vi "Begin.vi"(8 "error in":errorcluster) -> (0 "error out":errorcluster)   [LabVIEW 2016]
doc: "Called before other user functions, this VI is expected to open initial I/O refnums, load in file data, and do all program initialization. Notice that the <B>error out</B> terminal is simply used for data flow. Wiring it to other structures or subVIs ensures that this VI runs first."
uses:
  <vilib>/Rock Robotics/SystemInterfaces/DIO/FPGA_DIOPWMChannel.ctl
  <vilib>/Rock Robotics/WPI/SafetyOutput/WPI_SafetyOutputConfigMenu.ctl
  <vilib>/Rock Robotics/WPI/DriverStation/WPI_DriverStationRobotMode2.ctl
  <vilib>/Rock Robotics/WPI/Joystick/WPI_JoystickDeviceEnum.ctl
  <vilib>/Rock Robotics/SystemInterfaces/DIO/FPGA_DIOChannel.ctl
  <vilib>/Rock Robotics/WPI/RobotDrive/WPI_RobotDriveOpen2MotorWithTalon.vi
  Robot Global Data.vi
  <vilib>/Rock Robotics/Network Tables/NT Write String Array.vi
  <vilib>/Rock Robotics/WPI/Ultrasonic/WPI_SonarSRF04DigitalOpen.vi
  <vilib>/Rock Robotics/WPI/Ultrasonic/WPI_SonarSRF04DigitalRefNum Registry Set.vi
  Globals/Globals.vi
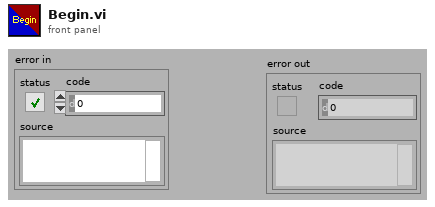
[diagram p1: front panel]
types:
  T1 = typedef "FPGA_DIOChannel.ctl" = enum8{"DIO 0", "DIO 1", "DIO 2", "DIO 3", "DIO 4", "DIO 5", "DIO 6", "DIO 7", "DIO 8", "DIO 9", "DIO MXP 0", "DIO MXP 1", "DIO MXP 2", "DIO MXP 3", "DIO MXP 4", "DIO MXP 5", "DIO MXP 6", "DIO MXP 7", "DIO MXP 8", "DIO MXP 9", "DIO MXP 10", "DIO MXP 11", "DIO MXP 12", "DIO MXP 13", "DIO MXP 14", "DIO MXP 15", "SPI Port CS1", "SPI Port CS2", "SPI Port CS3", "SPI Port MISO", "SPI Port MOSI", "Invalid"}
  T2 = typedef "FPGA_DIOPWMChannel.ctl" = enum8{"PWM 0", "PWM 1", "PWM 2", "PWM 3", "PWM 4", "PWM 5", "PWM 6", "PWM 7", "PWM 8", "PWM 9", "PWM MXP 0", "PWM MXP 1", "PWM MXP 2", "PWM MXP 3", "PWM MXP 4", "PWM MXP 5", "PWM MXP 6", "PWM MXP 7", "PWM MXP 8", "PWM MXP 9", "Invalid"}
  T3 = typedef "WPI_JoystickDeviceEnum.ctl" = enum16{"USB 0", "USB 1", "USB 2", "USB 3", "USB 4", "USB 5"}
  T4 = typedef "WPI_DriverStationRobotMode2.ctl" = enum16{"Autonomous Disabled", "Autonomous Enabled", "Teleop Disabled", "Teleop Enabled", "Disconnected", "Finish", "Test Disabled", "Test Enabled", "Emergency Stopped"}
  T5 = typedef "WPI_SafetyOutputConfigMenu.ctl" = enum16{"Enable", "Disable"}
  T6 = typedef "WPI_UltrasonicDeviceRef.ctl" = cluster{"DevStatus":errorcluster, "Ping Channel":T1, "Echo Channel":T1, "CntIndex":T7}
  T7 = typedef "FPGA_CounterCtrSystemIndex.ctl" = enum8{"Ctr 0", "Ctr 1", "Ctr 2", "Ctr 3", "Ctr 4", "Ctr 5", "Ctr 6", "Ctr 7", "Invalid"}
  T8 = typedef "WPI_JoystickDevRef.ctl" = cluster{"Device":T3}
  T9 = typedef "WPI_RobotDriveDevRef.ctl" = cluster{"DevStatus":errorcluster, "Motors[]":T10[], "Square Inputs":bool, "Max Output":dbl}
  T10 = typedef "WPI_MotorControlDeviceRef.ctl" = cluster{"DeviceStatus":errorcluster, "Type":T11, "PWM":cluster{"PWM Channel":T2, "DeadBand":T12}, "CAN":cluster{"Device Number":u8, "SetOutput VI Ref":variant, "GetOutput VI Ref":variant, "Enable VI Ref":variant, "Disable VI Ref":variant, "Data":variant}, "Invert":bool}
  T11 = typedef "WPI_MotorControlType.ctl" = enum16{"PWM", "CAN"}
  T12 = typedef "WPI_PWMDeadband.ctl" = cluster{"Name":string, "maxPositivePwm":i32, "minPositivePwm":i32, "centerPwm":i32, "maxNegativePwm":i32, "minNegativePwm":i32, "angularRange":u16}
  T13 = typedef "WPI_ServoDeviceRef.ctl" = cluster{"DeviceStatus":errorcluster, "PWM Channel":T2, "DeadBand":T12}
  T14 = typedef "WPI_DigitalOutputDevRef.ctl" = cluster{"DIO Channel":T1, "DevStatus":errorcluster}
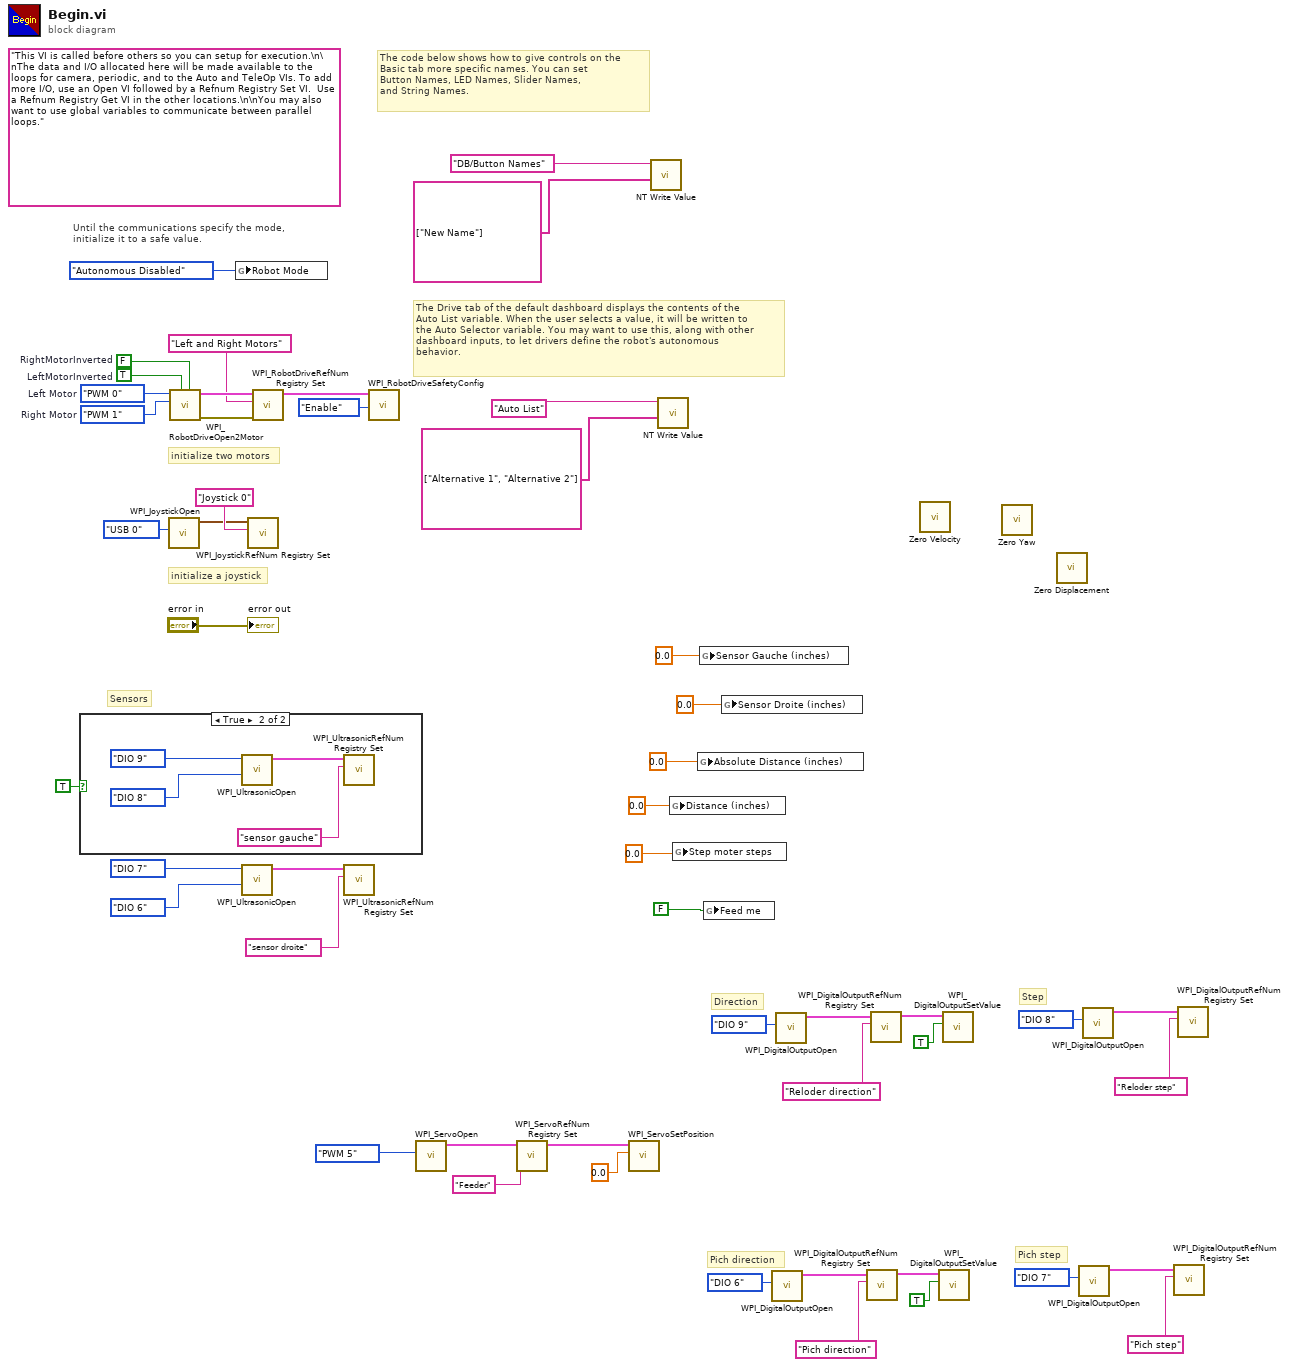
[diagram p0: block diagram]
diagram:
  (unwired) "This VI is called before others so you can setup for execution.\n\nThe data and I/O allocated here will be made available to the loops for camera, periodic, and to the Auto and TeleOp VIs. To add more I/O, use an Open VI followed by a Refnum Registry Set VI.  Use a Refnum Registry Get VI in the other locations.\n\nYou may also want to use global variables to communicate between parallel loops."
  w44 = FPGA_DIOPWMChannel."PWM 1"  # Right Motor
  w45 = FPGA_DIOPWMChannel."PWM 0"  # Left Motor
  w49 = TRUE  # LeftMotorInverted
  w50 = FALSE  # RightMotorInverted
  # "Pich direction"
  # "Pich step"
  # "Direction"
  # "Step"
  # "Sensors"
  # "The Drive tab of the default dashboard displays the contents of the\nAuto List variable. When the user selects a value, it will be written to\nthe Auto Selector variable. You may want to use this, along with other\ndashboard inputs, to let drivers define the robot's autonomous\nbehavior."
  # "The code below shows how to give controls on the\nBasic tab more specific names. You can set\nButton Names, LED Names, Slider Names,\nand String Names."
  # "initialize a joystick"
  # "Until the communications specify the mode,\ninitialize it to a safe value."
  # "initialize two motors"
  n1 = case shown="True" TRUE {
    frame False {
    }
    frame True {
      n2 = call-poly <vilib>:"WPI_UltrasonicOpen.vi"("Echo DIO Channel"=FPGA_DIOChannel."DIO 8", "Ping DIO Channel"=FPGA_DIOChannel."DIO 9") -> ("SonarSRF04DevRef"=w52:T6)  [unwired: 8 in, 1 out]
      n3 = call-poly <vilib>:"WPI_UltrasonicRefNum Registry Set.vi"("refnum name"="sensor gauche", "SonarSRF04DevRef"=w52) -> ()  [unwired: 8 in, 2 out]
    }
  }
  n4 = call <vilib>:"WPI_JoystickOpen.vi"("JoystickDevice"=WPI_JoystickDeviceEnum."USB 0") -> ("JoystickDevRef"=w39:T8)  [unwired: 10 in]
  n5 = call-poly <vilib>:"WPI_RobotDriveOpen2Motor.vi"("Right Motor Inverted"=w50, "Left Motor Inverted"=w49, "Right Motor"=w44, "Left Motor"=w45) -> ("error out"=w46:errorcluster, "RobotDriveDevRef"=w48:T9)  [unwired: 1 in, 5 out]
  n6 = global write "Robot Global Data.vi" "Robot Mode"(WPI_DriverStationRobotMode2."Autonomous Disabled" ("Robot Mode")) -> ()
  n7 = call-poly <vilib>:"WPI_UltrasonicOpen.vi"("Echo DIO Channel"=FPGA_DIOChannel."DIO 6", "Ping DIO Channel"=FPGA_DIOChannel."DIO 7") -> ("SonarSRF04DevRef"=w31:T6)  [unwired: 8 in, 1 out]
  n8 = call <vilib>:"WPI_JoystickRefNum Registry Set.vi"("refnum name"="Joystick 0", "JoystickDevRef"=w39) -> ()  [unwired: 8 in, 2 out]
  n9 = call <vilib>:"WPI_RobotDriveRefNum Registry Set.vi"("error in (no error)"=w46, "refnum name"="Left and Right Motors", "RobotDriveDevRef"=w48) -> ("RobotDriveDevRef"=w43:T9)  [unwired: 1 in, 7 out]
  n10 = call-poly <vilib>:"WPI_UltrasonicRefNum Registry Set.vi"("refnum name"="sensor droite", "SonarSRF04DevRef"=w31) -> ()  [unwired: 8 in, 2 out]
  n11 = call <vilib>:"WPI_RobotDriveSafetyConfig.vi"("mode"=WPI_SafetyOutputConfigMenu."Enable", "RobotDriveDevRef"=w43) -> ()  [unwired: 8 in, 2 out]
  n12 = call <vilib>:"WPI_ServoOpen.vi"("PWM Channel"=FPGA_DIOPWMChannel."PWM 5") -> ("ServoDeviceRef"=w14:T13)  [unwired: 9 in, 1 out]
  n13 = call <vilib>:"WPI_ServoRefNum Registry Set.vi"("refnum name"="Feeder", "ServoDeviceRef"=w14) -> ("ServoDeviceRef"=w13:T13)  [unwired: 8 in, 1 out]
  n14 = call <vilib>:"WPI_ServoSetPosition.vi"("Position"=0.0, "ServoDeviceRef"=w13) -> ()  [unwired: 8 in, 2 out]
  n15 = call-poly <vilib>:"NT Write Value.vi"("String Array"=string[] ["New Name"], "Name"="DB/Button Names") -> ()  [unwired: 9 in, 1 out]
  n16 = call-poly <vilib>:"NT Write Value.vi"("String Array"=string[] ["Alternative 1", "Alternative 2"], "Name"="Auto List") -> ()  [unwired: 9 in, 1 out]
  n17 = global write "Globals.vi" "Distance (inches)"(0.0 ("Sensor Gauche (inches)")) -> ()
  n18 = global write "Globals.vi" "Step moter steps"(0.0) -> ()
  n19 = global write "Globals.vi" "Absolute Distance (inches)"(0.0 ("Sensor Gauche (inches)")) -> ()
  n20 = global write "Globals.vi" "Sensor Gauche (inches)"(0.0 ("Sensor Gauche (inches)")) -> ()
  n21 = global write "Globals.vi" "Feed me"(FALSE ("Feed me")) -> ()
  n22 = global write "Globals.vi" "Sensor Droite (inches)"(0.0 ("Sensor Gauche (inches)")) -> ()
  n23 = call <vilib>:"WPI_DigitalOutputOpen.vi"("DIO Channel"=FPGA_DIOChannel."DIO 6") -> ("DigitalOutputDevRef"=w4:T14)  [unwired: 9 in, 1 out]
  n24 = call <vilib>:"WPI_DigitalOutputOpen.vi"("DIO Channel"=FPGA_DIOChannel."DIO 9") -> ("DigitalOutputDevRef"=w18:T14)  [unwired: 9 in, 1 out]
  n25 = call <vilib>:"WPI_DigitalOutputRefNum Registry Set.vi"("refnum name"="Pich direction", "DigitalOutputDevRef"=w4) -> ("DigitalOutputDevRef"=w2:T14)  [unwired: 8 in, 1 out]
  n26 = call <vilib>:"WPI_DigitalOutputRefNum Registry Set.vi"("refnum name"="Reloder direction", "DigitalOutputDevRef"=w18) -> ("DigitalOutputDevRef"=w16:T14)  [unwired: 8 in, 1 out]
  n27 = call <vilib>:"Zero Velocity.vi"() -> ()  [unwired: 12 in]
  n28 = call <vilib>:"WPI_DigitalOutputSetValue.vi"("Value"=TRUE, "DigitalOutputDevRef"=w2) -> ()  [unwired: 8 in, 2 out]
  n29 = call <vilib>:"WPI_DigitalOutputSetValue.vi"("Value"=TRUE, "DigitalOutputDevRef"=w16) -> ()  [unwired: 8 in, 2 out]
  n30 = call <vilib>:"Zero Yaw.vi"() -> ()  [unwired: 12 in]
  n31 = call <vilib>:"Zero Displacement.vi"() -> ()  [unwired: 12 in]
  n32 = call <vilib>:"WPI_DigitalOutputOpen.vi"("DIO Channel"=FPGA_DIOChannel."DIO 7") -> ("DigitalOutputDevRef"=w7:T14)  [unwired: 9 in, 1 out]
  n33 = call <vilib>:"WPI_DigitalOutputOpen.vi"("DIO Channel"=FPGA_DIOChannel."DIO 8") -> ("DigitalOutputDevRef"=w21:T14)  [unwired: 9 in, 1 out]
  n34 = call <vilib>:"WPI_DigitalOutputRefNum Registry Set.vi"("refnum name"="Pich step", "DigitalOutputDevRef"=w7) -> ()  [unwired: 8 in, 2 out]
  n35 = call <vilib>:"WPI_DigitalOutputRefNum Registry Set.vi"("refnum name"="Reloder step", "DigitalOutputDevRef"=w21) -> ()  [unwired: 8 in, 2 out]
  "error out" <- "error in"
